vi "CheckIO.vi"(10 "IONum":i32, 11 "PlatformNum":i32) -> ()   [LabVIEW 2011]
uses:
  API/API DYM.lvlib
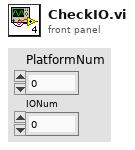
[diagram p1: front panel]
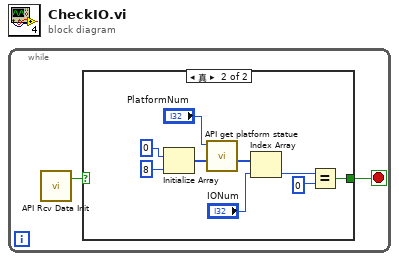
[diagram p0: block diagram]
diagram:
  n1 = while {
    stop <- w1 stop-if-true
    n2 = call "API Rcv Data Init.vi"() -> ("RTV"=w2:bool)  [unwired: 2 in, 1 out]
    n3 = case shown="真" w2 {
      selector: w2 -> [w3 _]
      tunnel: [w3 w4] -> w1
      frame False {
      }
      frame True {
        n4 = Initialize Array(0 ("元素"), 8 ("维数大小")) -> (w9:i32[])
        n5 = call "API get platform statue.vi"("platformStatue input"=w9, "PlatformNum"="PlatformNum") -> ("platformStatue output"=w8:i32[])  [unwired: 8 in, 1 out]
        n6 = Index Array(array=w8, index="IONum") -> (element=w6:i32)
        n7 = Equal?(x=w6, y=0) -> (x = y?=w4:bool)
      }
    }
  }
